vi "BuildMsg.vi"(7 "BuildType":T1 items=["simple", "Dialog", "PVUpdate", "Dialog&PV"], 8 "error in (no error)":errorcluster, 9 "ProgressBarCluster":T2, 10 "Msg to be build":string, 11 "CS++MessageMakerMain in":refnum<class "CS++MessageMakerMain.lvclass">) -> (0 "error out":errorcluster, 3 "CS++MessageMakerMain out":refnum<class "CS++MessageMakerMain.lvclass">)   [LabVIEW 2014, in "CS++MessageMakerMain.lvlib" / "CS++MessageMakerMain.lvclass"]
doc: "Passes the Build Message Command to the specific Actor Instance."
uses:
  CS++MessageMakerMain.lvclass
  BuildType.ctl
  CS++MessageMakerMain.lvclass/CS++MessageMakerMain.ctl
  CSPP_Actor/CS++Actor.lvclass/CS++Actor.ctl
  CSPP_Actor/CS++Actor.lvclass
  CSPP_MessageMaker_Utilities/CS++MessagemakerUtilities.lvlib
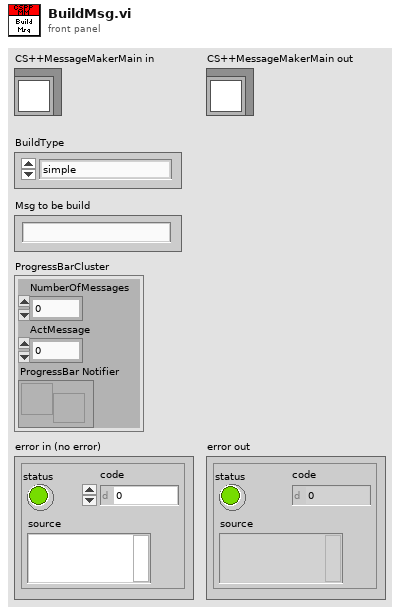
[diagram p1: front panel]
types:
  T1 = typedef "CS++MessageMakerMain.lvlib/CS++MessageMakerMain.lvclass/BuildType.ctl" = u16
  T2 = cluster{"NumberOfMessages":u16, "ActMessage":u16, "ProgressBar Notifier":refnum<notifier>}
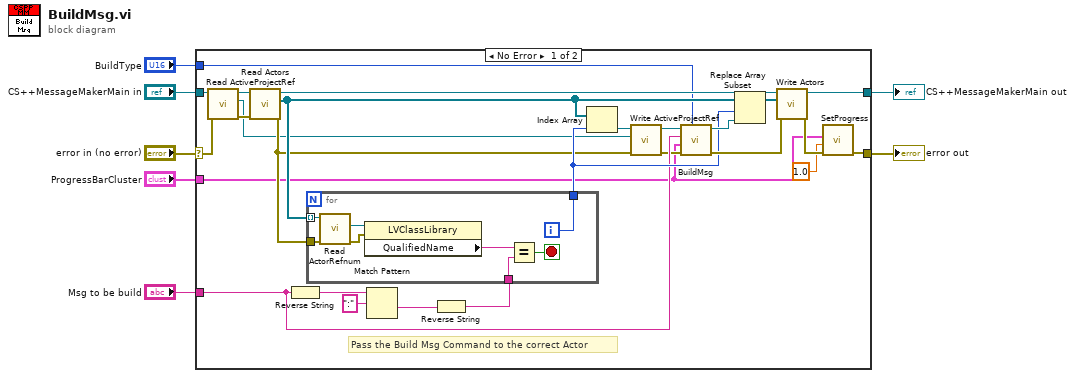
[diagram p0: block diagram]
diagram:
  n1 = case shown="No Error" "error in (no error)" {
    selector: "error in (no error)" -> [w14 w43]
    tunnel: [w11 w43] -> w6
    tunnel: [w31 w42] -> w4
    tunnel: "CS++MessageMakerMain in" -> [w16 w42]
    tunnel: "Msg to be build" -> [w22 _]
    tunnel: "ProgressBarCluster" -> [w9 _]
    tunnel: "BuildType" -> [w8 _]
    frame No Error {
      # "Pass the Build Msg Command to the correct Actor"
      n2 = call "Read ActiveProjectRef.vi"("error in (no error)"=w14, "CS++MessageMakerMain in"=w16) -> ("error out"=w15:errorcluster, "ActiveProjectRef"=w13:refnum<vi>, "CS++MessageMakerMain out"=w17:refnum<class "CS++MessageMakerMain.lvclass">)  [unwired: 7 in]
      n3 = call "Read Actors.vi"("error in (no error)"=w15, "CS++MessageMakerMain in"=w17) -> ("error out"=w18:errorcluster, "Actors"=w28:refnum<class "CS++Actor.lvclass">[], "CS++MessageMakerMain out"=w33:refnum<class "CS++MessageMakerMain.lvclass">)  [unwired: 7 in]
      n4 = Reverse String(1:w22) -> (0:w27:string)
      n5 = Match Pattern(string=w27, regular expression=":") -> (after substring=w25:string)  [unwired: 1 in, 3 out]
      n6 = Reverse String(1:w25) -> (0:w24:string)
      n7 = for {
        tunnel: w28 -> [w41] mode=indexing
        tunnel: w18 -> [w40]
        tunnel: w24 -> [w36]
        tunnel: [w34] -> w26
        i -> [w34]
        stop <- w35 stop-if-true
        n8 = call "Read ActorRefnum.vi"("error in (no error)"=w40, "CS++Actor in"=w41) -> ("error out"=w38:errorcluster, "ActorRefnum"=w39:refnum<vi>)  [unwired: 7 in, 1 out]
        n9 = property class="LVClassLibrary"(reference=w39, error in=w38) -> ("QualifiedName"=w37:string)  [unwired: 2 out]
        n10 = Equal?(x=w37, y=w36) -> (x = y?=w35:bool)
      }
      n11 = Index Array(array=w28, index=w26) -> (element=w20:refnum<class "CS++Actor.lvclass">)
      n12 = call "Write ActiveProjectRef.vi"("error in (no error)"=w18, "ActiveProjectRef"=w13, "CS++Actor in"=w20) -> ("error out"=w19:errorcluster, "CS++Actor out"=w21:refnum<class "CS++Actor.lvclass">)  [unwired: 7 in]
      n13 = call "BuildMsg.vi"("BuildType"=w8, "error in (no error)"=w19, "ProgressBarCluster"=w9, "Msg to be build"=w22, "CS++Actor in"=w21) -> ("error out"=w32:errorcluster, "CS++Actor out"=w29:refnum<class "CS++Actor.lvclass">)  [unwired: 5 in]
      n14 = Replace Array Subset(array=w28, new element=w29, index=w26) -> (w30:refnum<class "CS++Actor.lvclass">[])
      n15 = call "Write Actors.vi"("error in (no error)"=w32, "Actors"=w30, "CS++MessageMakerMain in"=w33) -> ("error out"=w12:errorcluster, "CS++MessageMakerMain out"=w31:refnum<class "CS++MessageMakerMain.lvclass">)  [unwired: 7 in]
      n16 = call "SetProgress.vi"("error in (no error)"=w12, "SubStep"=1.0, "ProgressBarCluster"=w9) -> ("error out"=w11:errorcluster)  [unwired: 8 in]
    }
    frame Error {
    }
  }
  "error out" <- w6
  "CS++MessageMakerMain out" <- w4
